vi "Library.vi"(5 "Config":refnum<class "TAF Proj Config.lvclass">, 7 "Lib Type":refnum<class "Lib.lvclass">, 8 "error in":errorcluster, 11 "Library Ref":refnum<vi>) -> (0 "error out":errorcluster, 3 "Lib out":refnum<class "Lib.lvclass">)   [LabVIEW 2021, in "TAF Proj Document Type.lvlib" / "Project Parser.lvlib"]
uses:
  <vilib>/Wovalab/AntiDoc/Document Type/Add-ons/LabVIEW TAF Project/Project Parser/Project Parser.lvlib
  <vilib>/Wovalab/AntiDoc/Document Type/Add-ons/LabVIEW TAF Project/Lib/Lib.lvclass
  <vilib>/Wovalab/AntiDoc/Document Type/Add-ons/LabVIEW TAF Project/TAF Proj Config/TAF Proj Config.lvclass
  <vilib>/Wovalab/AntiDoc/Document Type/Add-ons/LabVIEW TAF Project/Vi/Vi Info--cluster.ctl
  <vilib>/picture/picture.llb/imagedata.ctl
  <vilib>/Wovalab/AntiDoc/Document Type/Add-ons/LabVIEW TAF Project/Lib/Lib.lvclass/Lib.ctl
  <vilib>/Wovalab/AntiDoc/Document Type/Add-ons/LabVIEW TAF Project/Lib/Write Version.vi
  <vilib>/Wovalab/AntiDoc/Document Type/Add-ons/LabVIEW TAF Project/Lib/Write Nested Libraries.vi
  <vilib>/Wovalab/AntiDoc/Document Type/Add-ons/LabVIEW TAF Project/Vi/Vi.lvclass
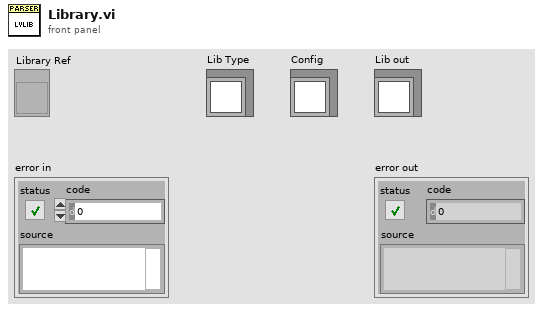
[diagram p1: front panel]
types:
  T1 = cluster{"Major":u16, "Minor":u16, "Fix":u16, "Build":u16}
  T2 = typedef "TAF Proj Document Type.lvlib/Vi.lvclass/Vi Info--cluster.ctl" = cluster{"Name":string, "Description":string, "Is Reentrant":bool, "Reentrancy Type":enum16{"Share clones between instances", "Preallocate clone for each instance"}, "Inline SubVI":bool, "Access Scope":enum32{"invalid scope", "public", "private", "protected", "community"}, "Conpane Image":T3}
  T3 = typedef "imagedata.ctl" = cluster{"image type":i32, "image depth":i32, "image":u8[], "mask":u8[], "colors":u32[], "Rectangle":cluster{"left":i16, "top":i16, "right":i16, "bottom":i16}}
  T4 = enum32{"invalid VI type", "Standard VI", "Control VI", "Global VI", "Polymorphic VI", "Configuration VI", "SubSystem", "Facade VI", "Method VI", "Statechart Diagram VI"}
  T5 = enum32{"invalid scope", "public", "private", "protected", "community"}
  T6 = enum16{"Share clones between instances", "Preallocate clone for each instance"}
  T7 = typedef "TAF Proj Document Type.lvlib/Lib.lvclass/Nested Lib Info--cluster.ctl" = cluster{"Name":string, "Type":string}
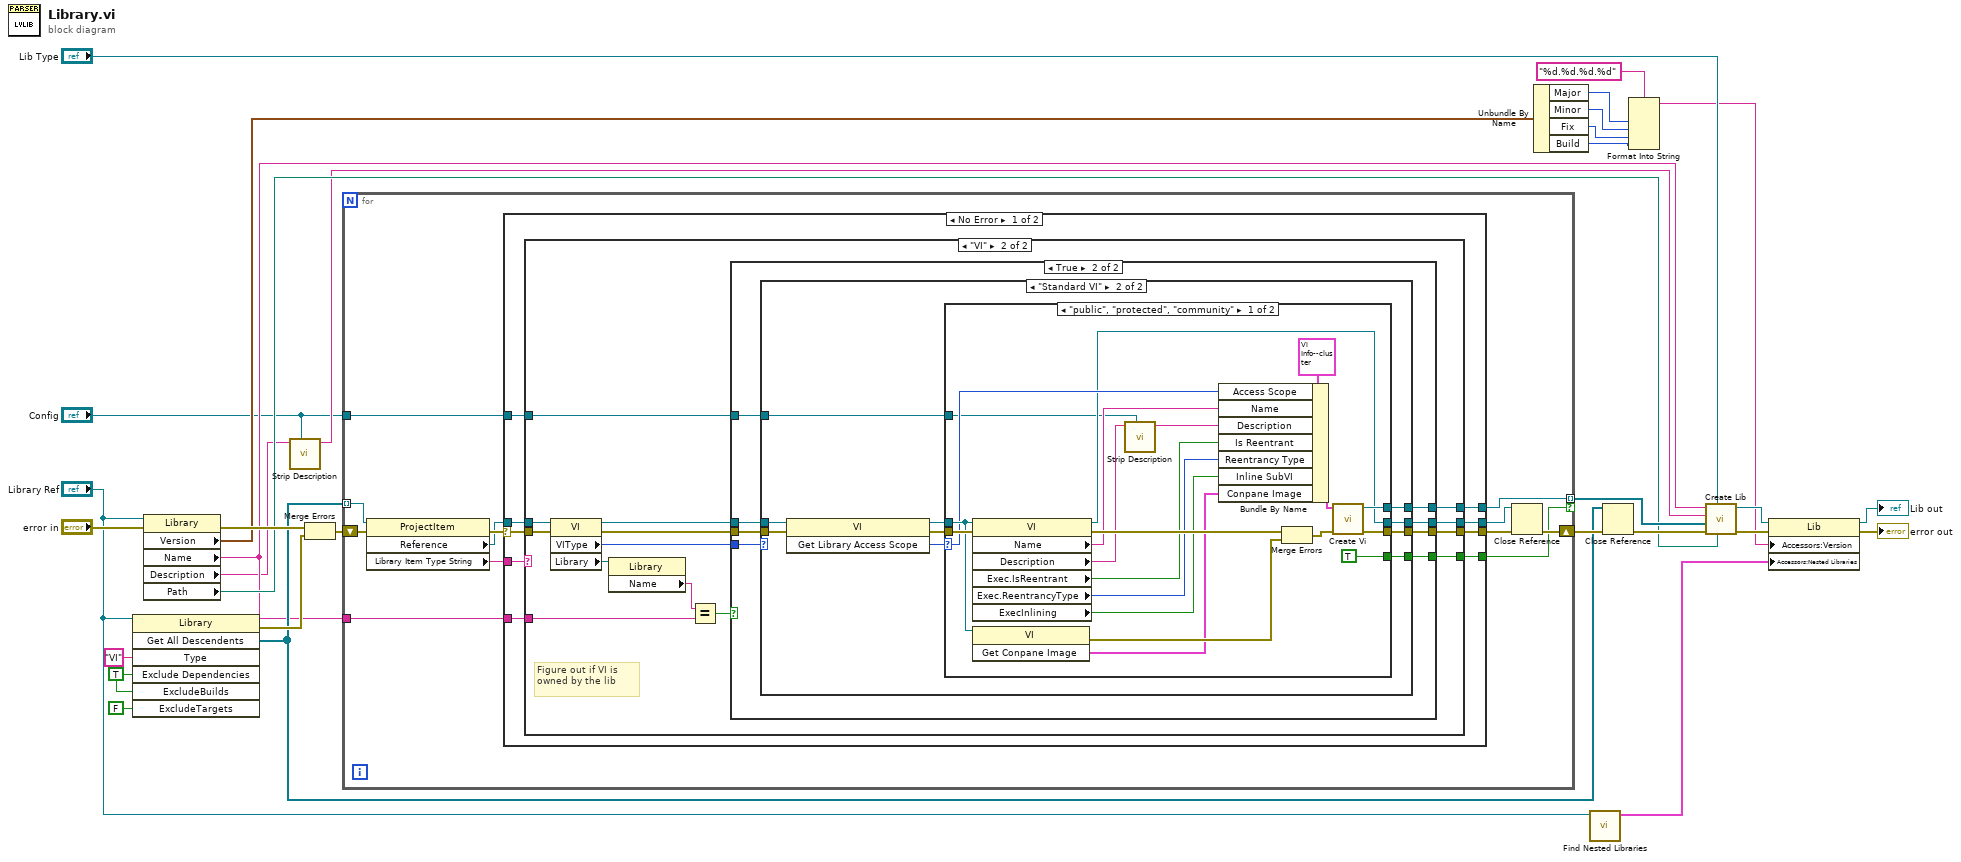
[diagram p0: block diagram]
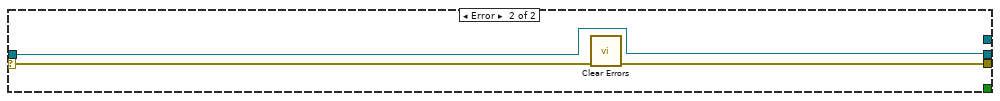
[diagram p6: hidden frame]
diagram:
  w20 = TRUE ("ExcludeDependencies")
  n1 = invoke class="Library" method="Get All Descendents"(reference="Library Ref", "Type"="VI", "Exclude Dependencies"=w20, "ExcludeBuilds"=w20, "ExcludeTargets"=FALSE) -> (error out=w29:errorcluster, "All Descendents"=w16:refnum<vi>[])  [unwired: 2 in, 5 out]
  n2 = property class="Library"(reference="Library Ref", error in="error in") -> (error out=w30:errorcluster, "Version"=w13:T1, "Name"=w4:string, "Description"=w3:string, "Path"=w18:path)  [unwired: 1 out]
  n3 = call <vilib>:"Strip Description.vi"("Config"="Config", "Description in"=w3) -> ("Description out"=w2:string)  [unwired: 9 in]
  n4 = Merge Errors(w30, w29) -> (w28:errorcluster)
  n5 = for {
    tunnel: w16 -> [w36] mode=indexing
    tunnel: [w38] -> w22 mode=indexing if=w37
    shift-right: [w40] -> w26
    shift-left: w28 -> [w42]
    tunnel: w4 -> [w32]
    tunnel: "Config" -> [w31]
    n6 = property class="ProjectItem"(reference=w36, error in=w42) -> (error out=w41:errorcluster, "Reference"=w35:refnum<vi>, "Library Item Type String"=w34:string)  [unwired: 1 out]
    n7 = case shown="No Error" w41 {
      selector: w41 -> [w51 w114]
      tunnel: w35 -> [w49 w112]
      tunnel: [w48 _] -> w38
      tunnel: [w47 _] -> w37
      tunnel: [w50 w113] -> w39
      tunnel: w34 -> [w46 _]
      tunnel: [w45 w112] -> w33
      tunnel: w32 -> [w44 _]
      tunnel: w31 -> [w43 _]
      frame No Error {
        n8 = case shown="\"VI\"" w46 {
          tunnel: w49 -> [w52 w61]
          tunnel: w51 -> [w53 w66]
          tunnel: [_ w64] -> w48
          tunnel: [_ w63] -> w47
          tunnel: [w53 w67] -> w50
          tunnel: [w52 w59] -> w45
          tunnel: w44 -> [_ w58]
          tunnel: w43 -> [_ w54]
          frame Default {
          }
          frame "VI" {
            # "Figure out if VI is owned by the lib"
            n9 = property class="VI"(reference=w61, error in=w66) -> (reference out=w60:refnum<vi>, error out=w65:errorcluster, "VIType"=w62:T4, "Library"=w56:refnum<vi>)
            n10 = property class="Library"(reference=w56) -> ("Name"=w55:string)  [unwired: 1 in, 2 out]
            n11 = Equal?(x=w55, y=w58) -> (x = y?=w57:bool)
            n12 = case shown="True" w57 {
              tunnel: [w69 w77] -> w67
              tunnel: w65 -> [w69 w76]
              tunnel: [_ w75] -> w64
              tunnel: [_ w74] -> w63
              tunnel: w62 -> [_ w73]
              tunnel: w60 -> [w68 w72]
              tunnel: [w68 w71] -> w59
              tunnel: w54 -> [_ w70]
              frame False {
                # "We list only VI directly owned by the lvlib"
              }
              frame True {
                n13 = case shown="\"Standard VI\"" w73 {
                  tunnel: w76 -> [w79 w89]
                  tunnel: [_ w84] -> w75
                  tunnel: [_ w83] -> w74
                  tunnel: [w79 w87] -> w77
                  tunnel: w72 -> [w78 w82]
                  tunnel: [w78 w81] -> w71
                  tunnel: w70 -> [_ w80]
                  frame Default {
                  }
                  frame "Standard VI" {
                    n14 = invoke class="VI" method="Get Library Access Scope"(reference=w82, error in=w89) -> (reference out=w85:refnum<vi>, error out=w88:errorcluster, "Get Library Access Scope"=w86:T5)  [unwired: 1 in]
                    n15 = case shown="\"public\", \"protected\", \"community\"" w86 {
                      selector: w86 -> [w96 _]
                      tunnel: w85 -> [w104 w110]
                      tunnel: w88 -> [w109 w111]
                      tunnel: [w103 _] -> w84
                      tunnel: [TRUE _] -> w83
                      tunnel: [w105 w111] -> w87
                      tunnel: [w93 w110] -> w81
                      tunnel: w80 -> [w90 _]
                      frame "public", "protected", "community" {
                        n16 = property class="VI"(reference=w104, error in=w109) -> (reference out=w93:refnum<vi>, error out=w108:errorcluster, "Name"=w99:string, "Description"=w92:string, "Exec.IsReentrant"=w98:bool, "Exec.ReentrancyType"=w97:T6, "ExecInlining"=w95:bool)
                        n17 = invoke class="VI" method="Get Conpane Image"(reference=w104) -> (error out=w107:errorcluster, "Get Conpane Image"=w94:T3)  [unwired: 2 in, 1 out]
                        n18 = call <vilib>:"Strip Description.vi"("Config"=w90, "Description in"=w92) -> ("Description out"=w91:string)  [unwired: 9 in]
                        n19 = Bundle By Name(cluster=T2 {"Name"="", "Description"="", "Is Reentrant"=FALSE, "Reentrancy Type"=enum."Share clones between instances", "Inline SubVI"=FALSE, "Access Scope"=enum."invalid scope", "Conpane Image"={"image type"=0, "image depth"=0, "image"=[], "mask"=[], "colors"=[], "Rectangle"={"left"=0, "top"=0, "right"=0, "bottom"=0}}} ("Vi Info"), "Access Scope"=w96, "Name"=w99, "Description"=w91, "Is Reentrant"=w98, "Reentrancy Type"=w97, "Inline SubVI"=w95, "Conpane Image"=w94) -> (w100:T2)
                        n20 = Merge Errors(w108, w107) -> (w106:errorcluster)
                        n21 = call <vilib>:"Create Vi.vi"("error in"=w106, "Vi Info"=w100) -> ("error out"=w105:errorcluster, "Vi out"=w103:refnum<class "Vi.lvclass">)  [unwired: 8 in]
                      }
                      frame "invalid scope", "private" {
                      }
                    }
                  }
                }
              }
            }
          }
        }
      }
      frame Error {
        n22 = call <vilib>:"Clear Errors.vi"("error in (no error)"=w114) -> ("error out"=w113:errorcluster)  [unwired: 5 in, 1 out]
      }
    }
    n23 = Close Reference(reference=w33, error in (no error)=w39) -> (error out=w40:errorcluster)
  }
  n24 = Unbundle By Name(w13) -> ("Major"=w12:u16, "Minor"=w11:u16, "Fix"=w10:u16, "Build"=w9:u16)
  n25 = call <vilib>:"Find Nested Libraries.vi"("Library Ref"="Library Ref") -> ("Nested Libraries"=w6:T7[])  [unwired: 10 in]
  n26 = Close Reference(reference=w16, error in (no error)=w26) -> (error out=w25:errorcluster)
  n27 = Format Into String(format string="%d.%d.%d.%d", w12, w11, w10, w9) -> (resulting string=w7:string)  [unwired: 2 in, 1 out]
  n28 = call <vilib>:"Create Lib.vi"("Path"=w18, "Lib Type"="Lib Type", "error in"=w25, "Vis"=w22, "Description"=w2, "Name"=w4) -> ("error out"=w24:errorcluster, "Lib out"=w15:refnum<class "Lib.lvclass">)  [unwired: 4 in]
  n29 = property class="Lib"(reference=w15, error in=w24, "Accessors:Version"=w7, "Accessors:Nested Libraries"=w6) -> (reference out=→"Lib out":refnum<class "Lib.lvclass">, error out=→"error out":errorcluster)
